vi "Index_Array.vi"() -> ()   [LabVIEW 2019]
panel:
  out "Last Value":dbl
  out "Array":dbl[](array[numeric])
  # "Index Array"
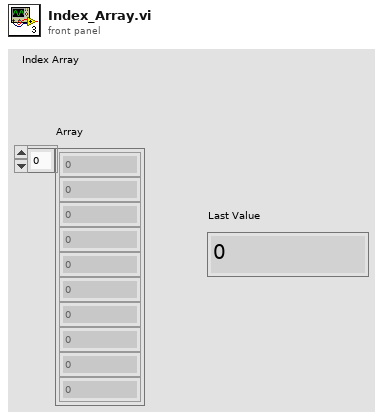
[diagram p1: front panel]
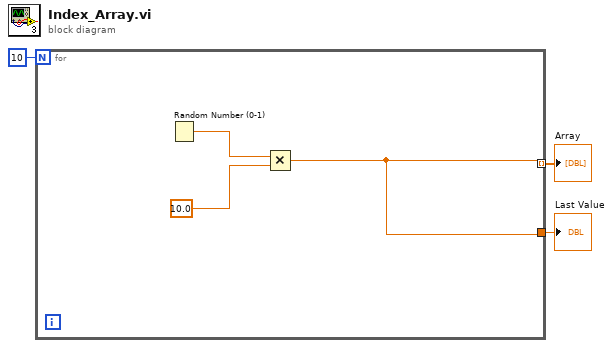
[diagram p0: block diagram]
diagram:
  n1 = for {
    N: 10 -> [_]
    tunnel: [w4] -> w2 mode=indexing
    tunnel: [w4] -> w1
    n2 = Random Number (0-1)() -> (number: 0 to 1=w5:dbl)
    n3 = Multiply(x=w5, y=10.0) -> (x*y=w4:dbl)
  }
  "Array" <- w2
  "Last Value" <- w1
